vi "Read Inputs from system.vi"(8 "error in":errorcluster, 11 "ExampleSequencer runtime in":refnum<class "ExampleSequencer runtime.lvclass">) -> (0 "error out":errorcluster, 2 "Inputs from system":T1, 3 "ExampleSequencer runtime out":refnum<class "ExampleSequencer runtime.lvclass">)   [LabVIEW 2017, in "ExampleSequencer runtime.lvclass"]
uses:
  ExampleSequencer runtime.lvclass
  configuration/input data indices.ctl
  ExampleSequencer runtime.lvclass/ExampleSequencer runtime.ctl
  configuration/ExampleSequencer configuration.lvclass
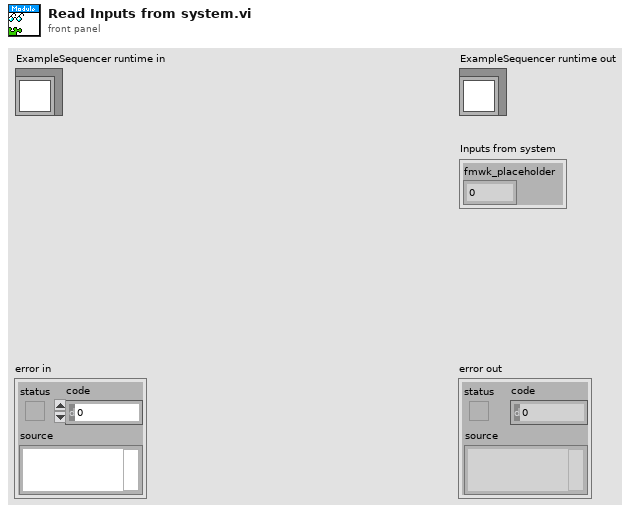
[diagram p1: front panel]
types:
  T1 = typedef "ExampleSequencer configuration.lvclass/input data indices.ctl" = cluster{"fmwk_placeholder":i32}
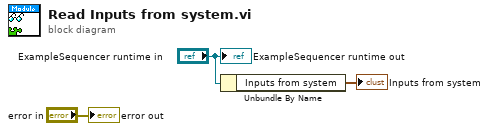
[diagram p0: block diagram]
diagram:
  n1 = Unbundle By Name("ExampleSequencer runtime in") -> ("Inputs from system"=→"Inputs from system":T1)
  "error out" <- "error in"
  "ExampleSequencer runtime out" <- "ExampleSequencer runtime in"
